vi "facade.vi"(0 "Data In":T13, 2 "Display State In":T3={"current frame index"=0, "number of images"=0, "ROI (frames)"={"ROI"=[]}, "control refs"={"frame"=refnum, "image"=refnum, "saveROIsButton"=refnum, "loadImageSwitch"=refnum, "loadROIsSwitch"=refnum, "saveROIsSwitch"=refnum, "loadImagePath"=refnum, "loadROIPath"=refnum, "redraw"=refnum}, "calibration"={"x"=0.0, "y"=0.0, "x unit"=enum."um", "y unit"=enum."um"}, "xpaths"={"x offset"="", "y offset"="", "z offset"=""}, "offset"=refnum, "XML description"="", "number of ROIs"=0.0, "ROI Tool Buttons Visible"={"Zoom Tool"=FALSE, "Selection Tool"=FALSE, "Pan Tool"=FALSE, "Point Tool"=FALSE, "Line Tool"=FALSE, "Rectangle Tool"=FALSE, "Rotated Rectangle Tool"=FALSE, "Polyline Tool"=FALSE, "Polygon Tool"=FALSE, "Freehand Tool"=FALSE, "Closed Freehand Tool"=FALSE, "Ellipse Tool"=FALSE, "Annulus Tool"=FALSE}, "ROI color"=0, "enable ROI numbering?"=FALSE, "selected path to save ROIs"=path "", "starting path"=path "", "loaded image path"=path "", "array of overlays"=[], "pointCollection"=refnum, "ROImode"=enum."IMAQROIs", "selected point ID"=0.0, "point radius"=0, "point colours"=[], "PlotAreaSize"={"Width"=0, "Height"=0}, "last action"=enum."not specified"} {"array of overlays"."overlay size" min=1}, 3 "Container State":T12, 5 "error in (no error)":errorcluster) -> (4 "error out":errorcluster, 6 "Data Out":T13, 7 "Display State Out":T3={"current frame index"=0, "number of images"=0, "ROI (frames)"={"ROI"=[]}, "control refs"={"frame"=refnum, "image"=refnum, "saveROIsButton"=refnum, "loadImageSwitch"=refnum, "loadROIsSwitch"=refnum, "saveROIsSwitch"=refnum, "loadImagePath"=refnum, "loadROIPath"=refnum, "redraw"=refnum}, "calibration"={"x"=0.0, "y"=0.0, "x unit"=enum."um", "y unit"=enum."um"}, "xpaths"={"x offset"="", "y offset"="", "z offset"=""}, "offset"=refnum, "XML description"="", "number of ROIs"=0.0, "ROI Tool Buttons Visible"={"Zoom Tool"=FALSE, "Selection Tool"=FALSE, "Pan Tool"=FALSE, "Point Tool"=FALSE, "Line Tool"=FALSE, "Rectangle Tool"=FALSE, "Rotated Rectangle Tool"=FALSE, "Polyline Tool"=FALSE, "Polygon Tool"=FALSE, "Freehand Tool"=FALSE, "Closed Freehand Tool"=FALSE, "Ellipse Tool"=FALSE, "Annulus Tool"=FALSE}, "ROI color"=0, "enable ROI numbering?"=FALSE, "selected path to save ROIs"=path "", "starting path"=path "", "loaded image path"=path "", "array of overlays"=[], "pointCollection"=refnum, "ROImode"=enum."IMAQROIs", "selected point ID"=0.0, "point radius"=0, "point colours"=[], "PlotAreaSize"={"Width"=0, "Height"=0}, "last action"=enum."not specified"} {"array of overlays"."overlay size" min=1}, 8 "Action":T2)   [LabVIEW 2010, in "XImage.xctl"]
uses:
  XImage.xctl
  data.ctl
  classes/ImageCollection/ImageCollection/ImageCollection.lvclass
  <vilib>/_xctls/Container State.ctl
  state.ctl
  classes/SpaceVector/SpaceVector/SpaceVector.lvclass
  classes/PointCollection/PointCollection/PointCollection.lvclass
  ROI_frames_cluster.ctl
  control_refs_cluster.ctl
  calibration_cluster.ctl
  enumerations/unit.ctl
  xpath_cluster.ctl
  overlays_cluster.ctl
  ROI_mode_enum.ctl
  last_action_enum.ctl
  <vilib>/_xctls/Action.ctl
  classes/Image/Image/Image.lvclass
  <vilib>/vision/Image Controls.llb/IMAQ Image.ctl
  <vilib>/Utility/inputDevices.llb/keyboardAcquire.vi
  <vilib>/Utility/inputDevices.llb/closeKeyboard.vi
  <vilib>/_xctls/XControlSupport.lvlib
panel:
  out "event case no.":i32
  in  "redraw":bool
  in  "savePointsButton":bool
  in  "loadPointsButton":bool
  in  "showHeaderButton":bool
  in  "loadROIPath":path caption="start path"
  in  "loadImagePath":path
  in  "loadROIsSwitch":bool=TRUE
  in  "saveROIsSwitch":bool=TRUE
  in  "loadImageSwitch":bool=TRUE
  out "progress bar":u8(slide) scale=0.0..100.0
  in  "loadROIsButton":bool
  in  "saveROIsButton":bool
  in  "loadImageButton":bool
  in  "frame":i32(slide) scale=0.0..10.0
  out "Image":T1(plugin-control)
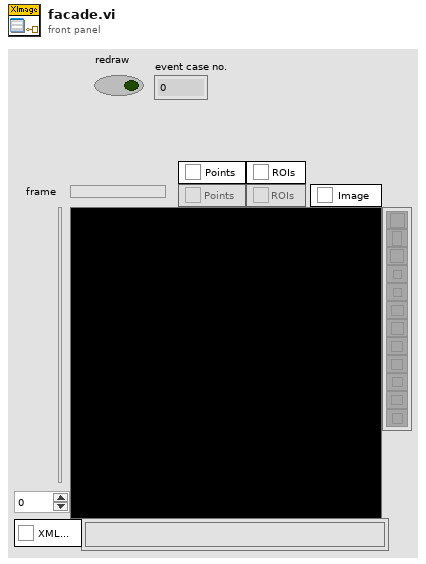
[diagram p1: front panel]
types:
  T1 = typedef "IMAQ Image.ctl" = refnum<image>
  T2 = typedef "XControlSupport.lvlib/Action.ctl" = cluster{"Data Changed?":bool, "State Changed?":bool, "Action Name":string}
  T3 = typedef "XImage.xctl/state.ctl" = cluster{"current frame index":i32, "number of images":i32, "ROI (frames)":T4, "control refs":T5, "calibration":T6, "xpaths":T8, "offset":refnum<class "SpaceVector.lvclass">, "XML description":string, "number of ROIs":dbl, "ROI Tool Buttons Visible":cluster{"Zoom Tool":bool, "Selection Tool":bool, "Pan Tool":bool, "Point Tool":bool, "Line Tool":bool, "Rectangle Tool":bool, "Rotated Rectangle Tool":bool, "Polyline Tool":bool, "Polygon Tool":bool, "Freehand Tool":bool, "Closed Freehand Tool":bool, "Ellipse Tool":bool, "Annulus Tool":bool}, "ROI color":u32, "enable ROI numbering?":bool, "selected path to save ROIs":path, "starting path":path, "loaded image path":path, "array of overlays":T9[], "pointCollection":refnum<class "PointCollection.lvclass">, "ROImode":T10, "selected point ID":dbl, "point radius":i32, "point colours":u32[], "PlotAreaSize":cluster{"Width":u32, "Height":u32}, "last action":T11}
  T4 = typedef "XImage.xctl/ROI_frames_cluster.ctl" = cluster{"ROI":cluster{"Global Rectangle":i32[], "Contours":cluster{"Contour Type":u32, "ROI Type":u32, "Points":i32[]}[]}[]}
  T5 = typedef "XImage.xctl/control_refs_cluster.ctl" = cluster{"frame":refnum<vi>, "image":refnum<vi>, "saveROIsButton":refnum<vi>, "loadImageSwitch":refnum<vi>, "loadROIsSwitch":refnum<vi>, "saveROIsSwitch":refnum<vi>, "loadImagePath":refnum<vi>, "loadROIPath":refnum<vi>, "redraw":refnum<vi>}
  T6 = typedef "XImage.xctl/calibration_cluster.ctl" = cluster{"x":dbl, "y":dbl, "x unit":T7, "y unit":T7}
  T7 = typedef "Image.lvclass/unit.ctl" = enum16{"um", "s"}
  T8 = typedef "XImage.xctl/xpath_cluster.ctl" = cluster{"x offset":string, "y offset":string, "z offset":string}
  T9 = typedef "XImage.xctl/overlays_cluster.ctl" = cluster{"overlay array":cluster{i32[][]}[], "overlay name":string, "color (red)":u32, "overlay size":i32, "overlay type":enum16{"crosshair", "circle"}}
  T10 = typedef "XImage.xctl/ROI_mode_enum.ctl" = enum16{"none", "IMAQROIs", "PointCollection"}
  T11 = typedef "XImage.xctl/last_action_enum.ctl" = enum16{"not specified", "image loaded", "frame changed", "ROIs changed"}
  T12 = typedef "XControlSupport.lvlib/Container State.ctl" = cluster{"Indicator?":bool, "Run Mode?":bool, " Refnum":refnum<vi>}
  T13 = typedef "XImage.xctl/data.ctl" = refnum<class "ImageCollection.lvclass">
  T14 = enum16{"0", "1", "2", "3", "4", "5", "6", "7", "8", "9", "A", "B", "C", "D", "E", "F", "G", "H", "I", "J", "K", "L", "M", "N", "O", "P", "Q", "R", "S", "T", "U", "V", "W", "X", "Y", "Z", "F1", "F2", "F3", "F4", "F5", "F6", "F7", "F8", "F9", "F10", "F11", "F12", "F13", "F14", "F15", "ADD", "BACK", "BACKSLASH", "CAPITAL", "COMMA", "DECIMAL", "DELETE", "DIVIDE", "DOWN", "END", "EQUALS", "ESCAPE", "GRAVE (`)", "HOME", "INSERT", "LBRACKET", "LCONTROL", "LEFT", "L ALT", "LSHIFT", "LWIN", "MINUS", "MULTIPLY", "NEXT", "NUMLOCK", "NUMPAD_0", "NUMPAD_1", "NUMPAD_2", "NUMPAD_3", "NUMPAD_4", "NUMPAD_5", "NUMPAD_6", "NUMPAD_7", "NUMPAD_8", "NUMPAD_9", "PAUSE", "PERIOD", "PRIOR (PG UP)", "RBRACKET", "RCONTROL", "RETURN", "RIGHT", "R ALT", "RSHIFT", "RWIN", "SCROLL", "SEMICOLON", "SLASH", "SPACE", "SUBTRACT", "TAB", "UP", "ENTER (num pad)", "' (quote)"}
  T15 = cluster{"Zoom Tool":bool, "Selection Tool":bool, "Pan Tool":bool, "Point Tool":bool, "Line Tool":bool, "Rectangle Tool":bool, "Rotated Rectangle Tool":bool, "Polyline Tool":bool, "Polygon Tool":bool, "Freehand Tool":bool, "Closed Freehand Tool":bool, "Ellipse Tool":bool, "Annulus Tool":bool}
  T16 = cluster{"Global Rectangle":i32[], "Contours":cluster{"Contour Type":u32, "ROI Type":u32, "Points":i32[]}[]}
  T17 = cluster{"Global Rectangle":i32[], "Contours":cluster{"Contour Type":u32, "ROI Type":u32, "Points":i32[]}[]}[]
  T18 = cluster{"Contour Type":u32, "ROI Type":u32, "Points":i32[]}[]
  T19 = enum8{"Enabled", "Disabled", "Disabled and Grayed Out"}
  T20 = typedef "Image Type" = u32
  T21 = enum16{"0", "1", "2", "3", "4", "5", "6", "7", "8", "9", "A", "B", "C", "D", "E", "F", "G", "H", "I", "J", "K", "L", "M", "N", "O", "P", "Q", "R", "S", "T", "U", "V", "W", "X", "Y", "Z", "F1", "F2", "F3", "F4", "F5", "F6", "F7", "F8", "F9", "F10", "F11", "F12", "F13", "F14", "F15", "ADD", "BACK", "BACKSLASH", "CAPITAL", "COMMA", "DECIMAL", "DELETE", "DIVIDE", "DOWN", "END", "EQUALS", "ESCAPE", "GRAVE (`)", "HOME", "INSERT", "LBRACKET", "LCONTROL", "LEFT", "L ALT", "LSHIFT", "LWIN", "MINUS", "MULTIPLY", "NEXT", "NUMLOCK", "NUMPAD_0", "NUMPAD_1", "NUMPAD_2", "NUMPAD_3", "NUMPAD_4", "NUMPAD_5", "NUMPAD_6", "NUMPAD_7", "NUMPAD_8", "NUMPAD_9", "PAUSE", "PERIOD", "PRIOR (PG UP)", "RBRACKET", "RCONTROL", "RETURN", "RIGHT", "R ALT", "RSHIFT", "RWIN", "SCROLL", "SEMICOLON", "SLASH", "SPACE", "SUBTRACT", "TAB", "UP", "ENTER (num pad)", "' (quote)"}[]
  T22 = typedef "LVRectTypeDef.ctl" = cluster{"left":i16, "top":i16, "right":i16, "bottom":i16}
  T23 = typedef "LVBoundsTypeDef.ctl" = cluster{"Width":u32, "Height":u32}
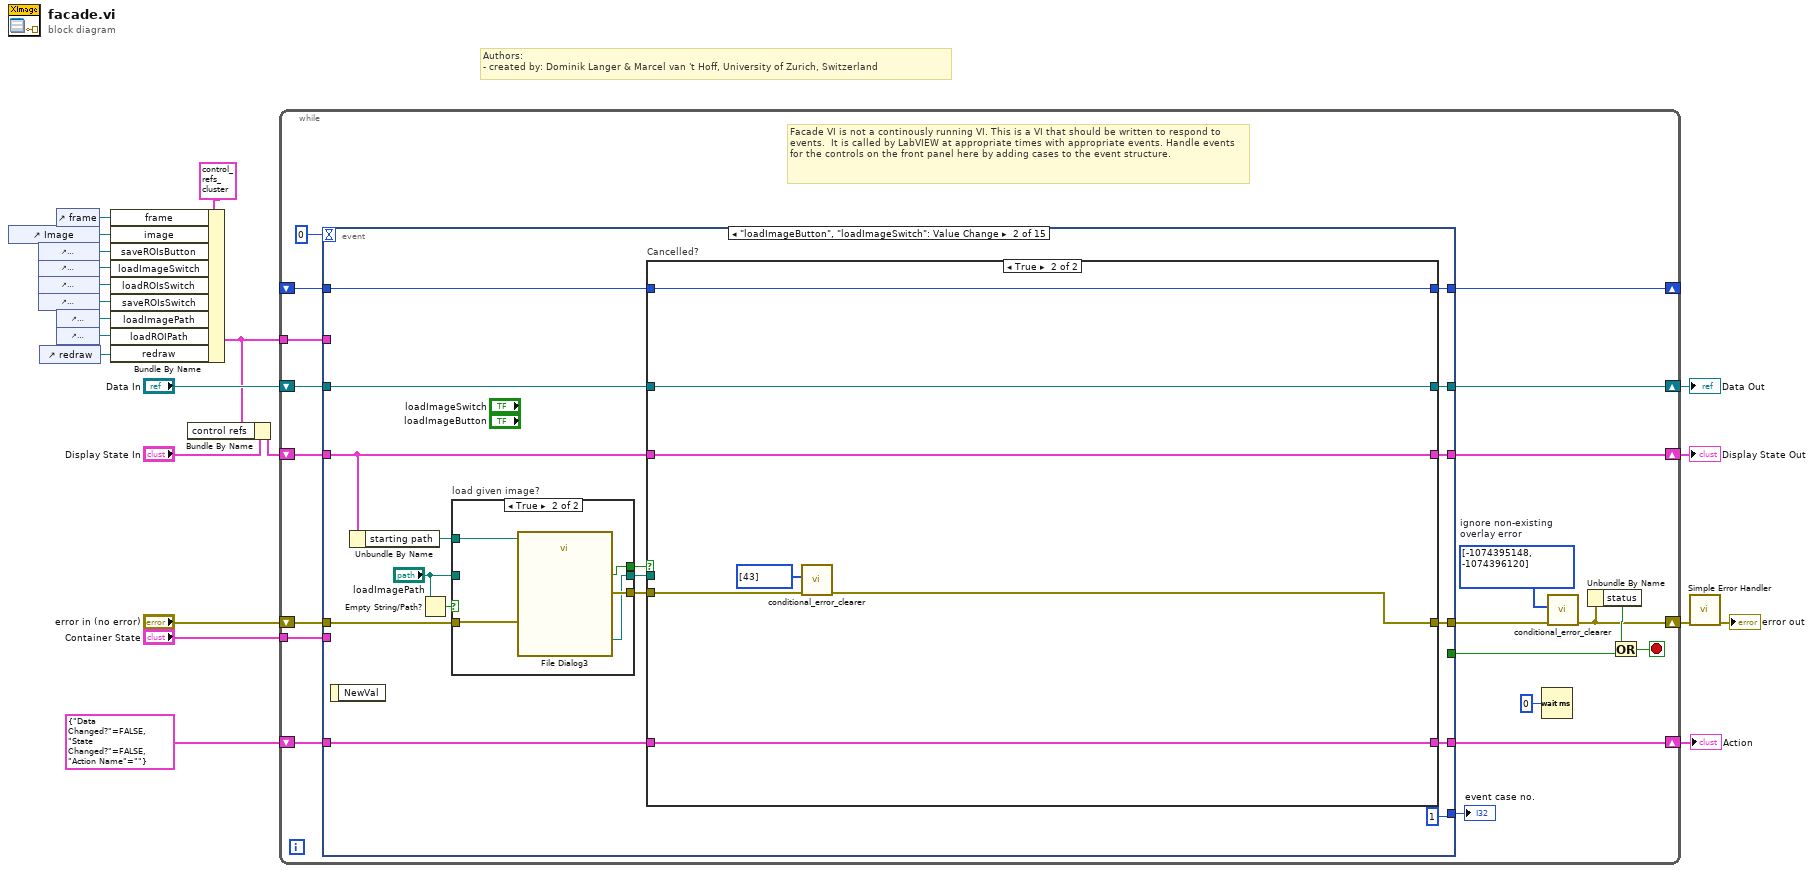
[diagram p0: block diagram]
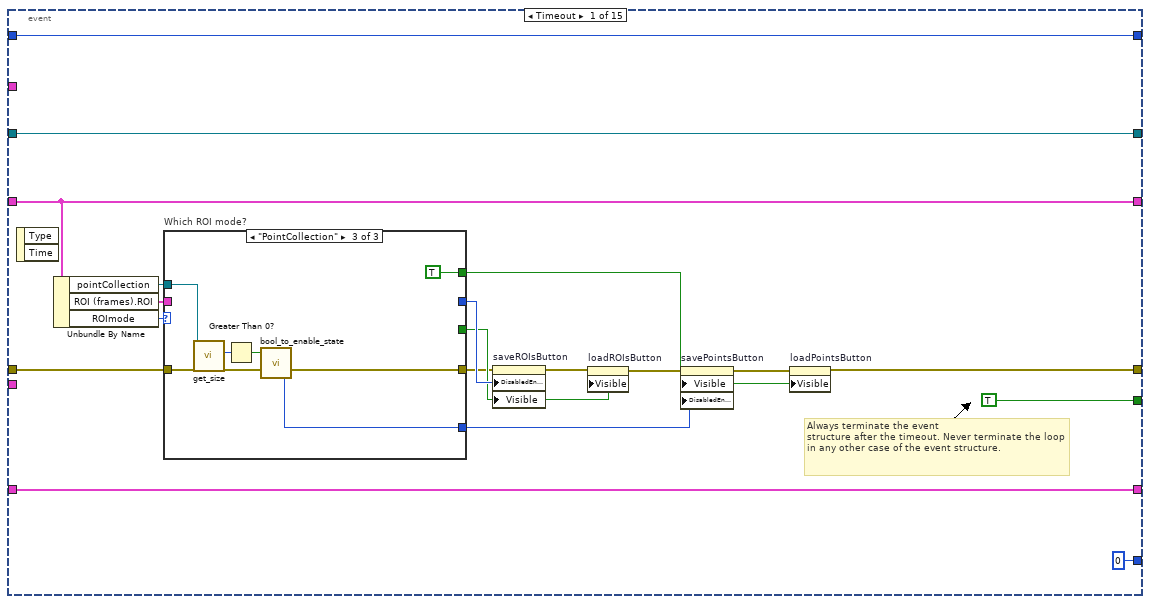
[diagram p2: hidden frame]
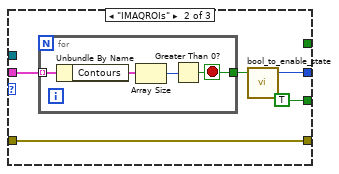
[diagram p4: hidden frame]
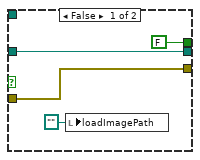
[diagram p5: hidden frame]
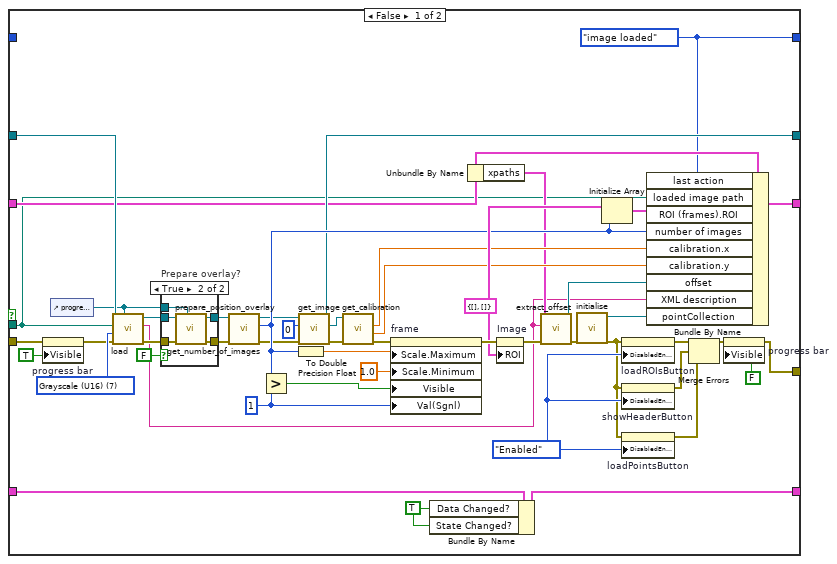
[diagram p6: hidden frame]
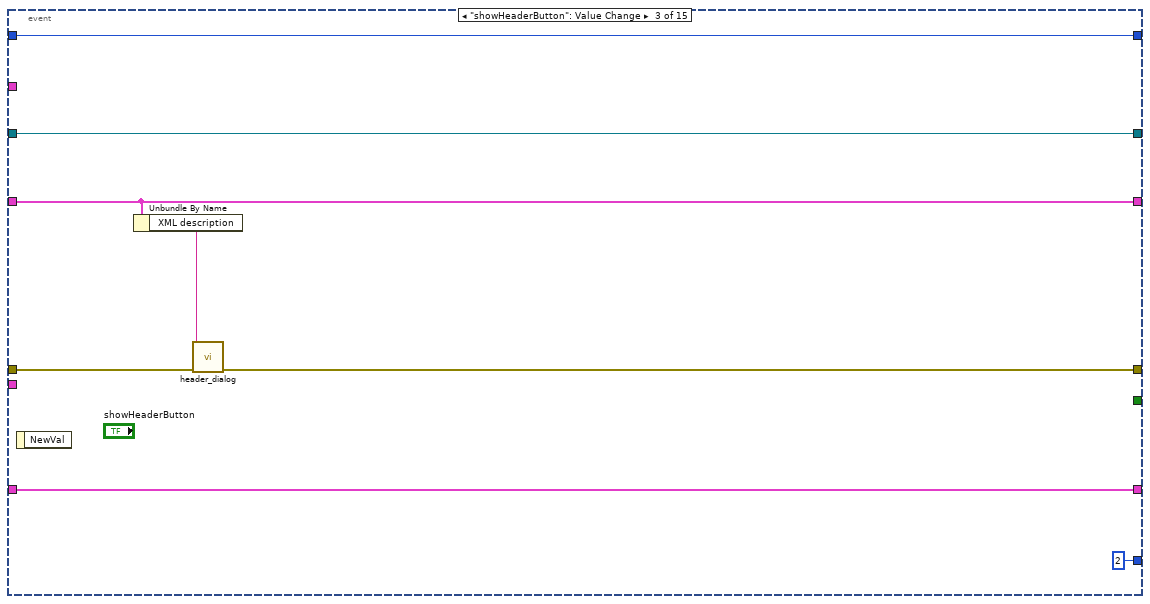
[diagram p8: hidden frame]
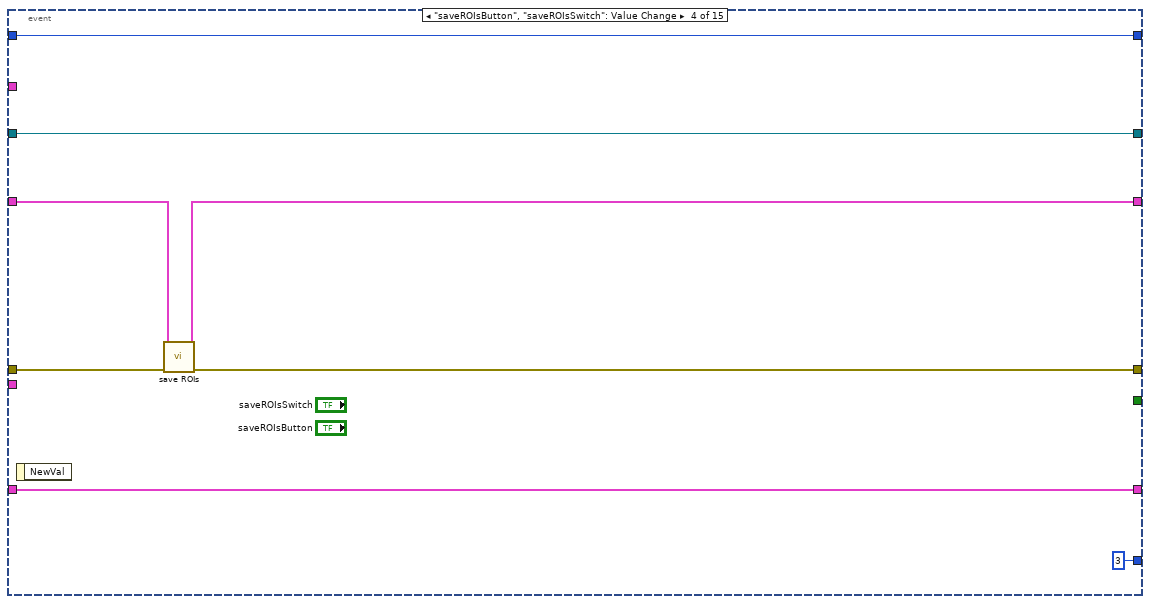
[diagram p9: hidden frame]
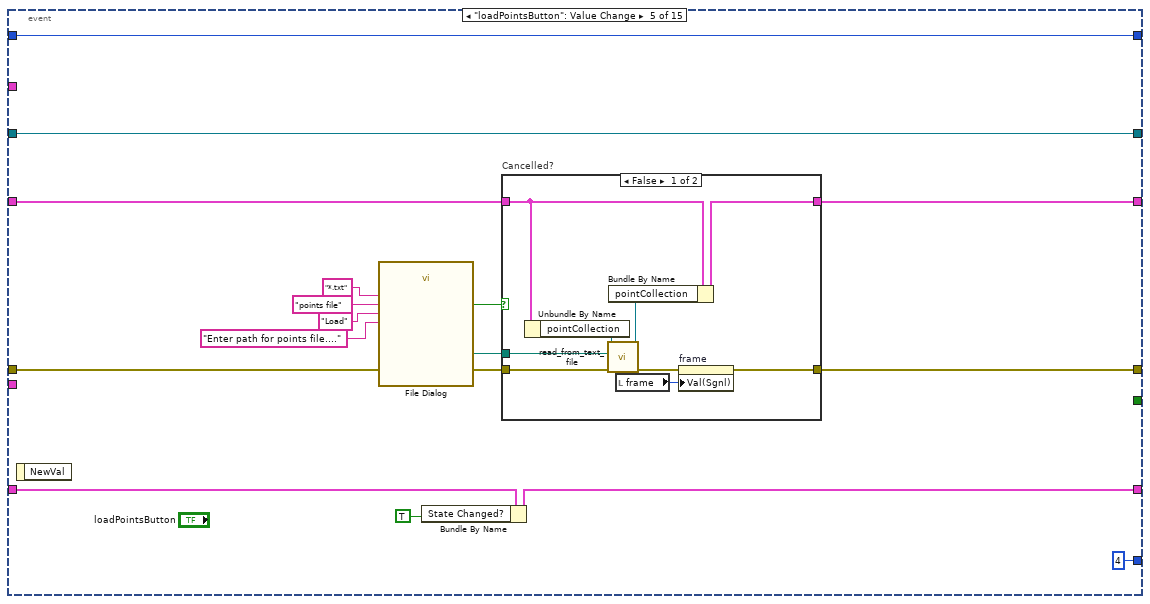
[diagram p10: hidden frame]
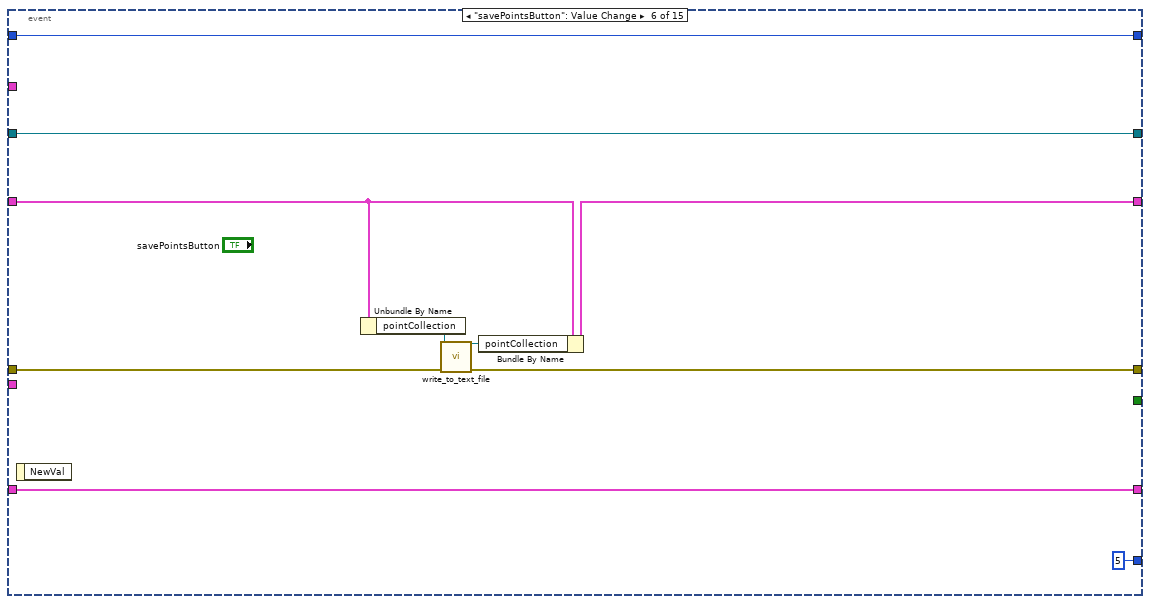
[diagram p12: hidden frame]
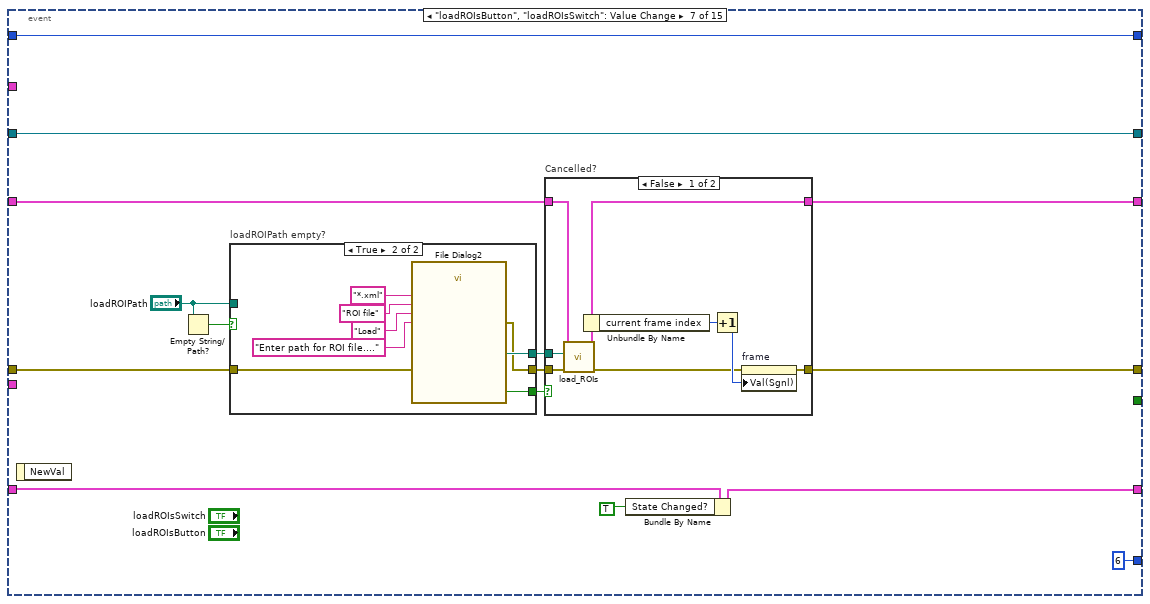
[diagram p13: hidden frame]
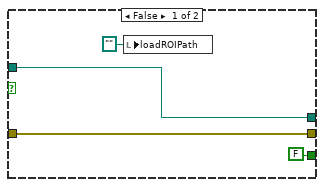
[diagram p14: hidden frame]
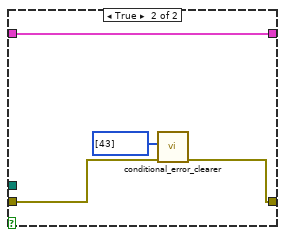
[diagram p15: hidden frame]
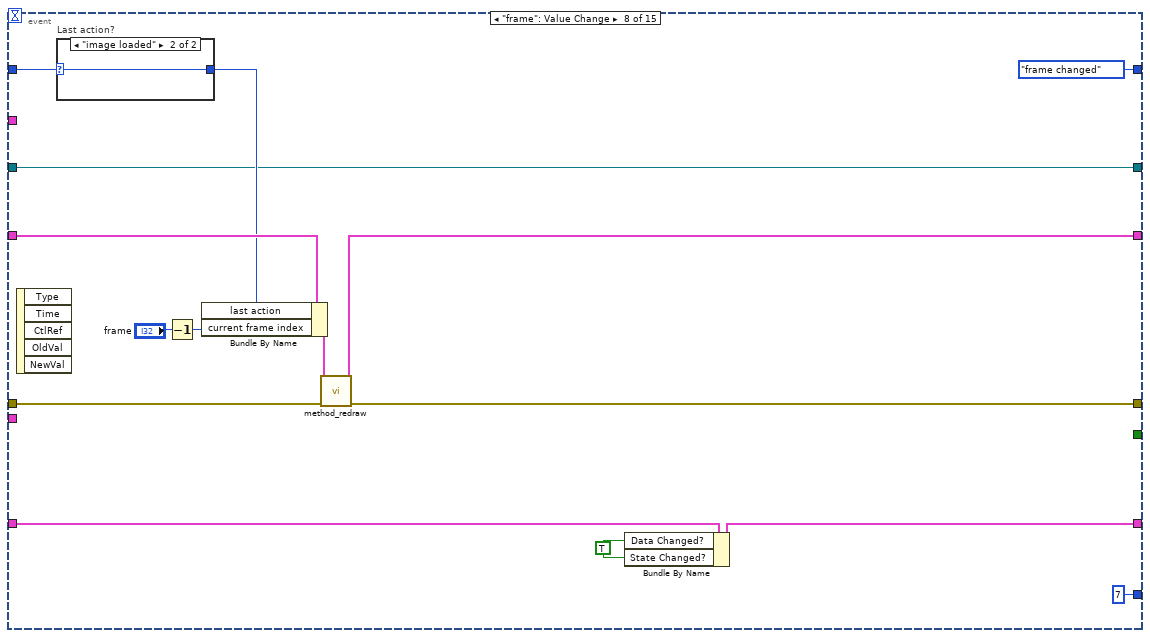
[diagram p16: hidden frame]
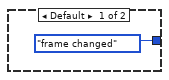
[diagram p17: hidden frame]
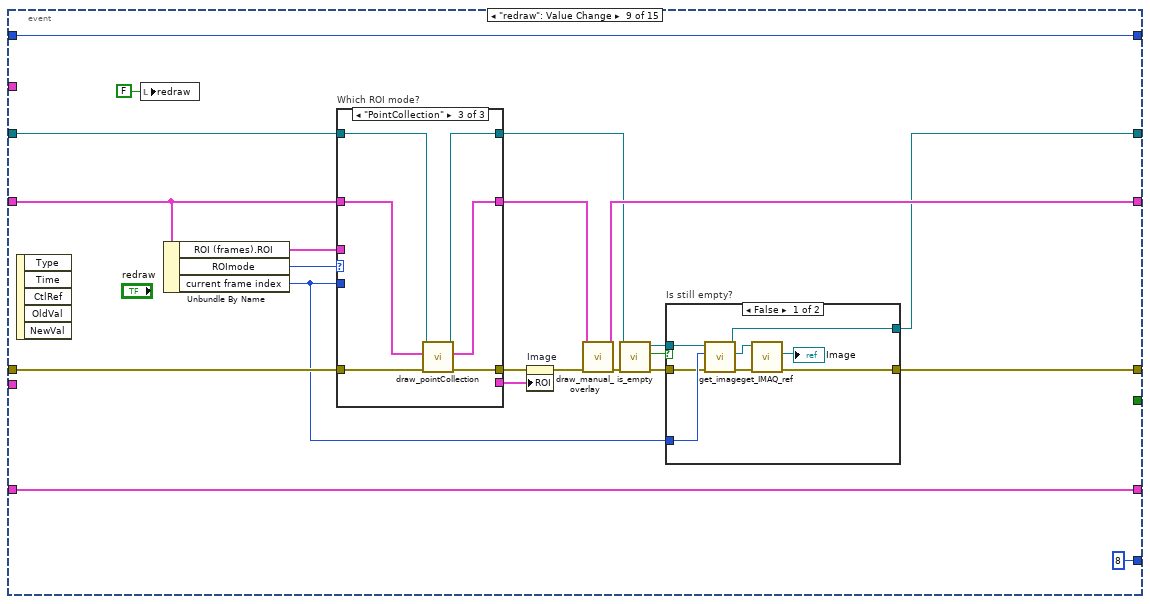
[diagram p18: hidden frame]
diagram:
  # "Authors: \n- created by: Dominik Langer & Marcel van 't Hoff, University of Zurich, Switzerland"
  n1 = control-ref of="Image"() -> (w8:refnum<vi>)
  n2 = control-ref of="saveROIsButton"() -> (w9:refnum<vi>)
  n3 = control-ref of="loadImageSwitch"() -> (w10:refnum<vi>)
  n4 = control-ref of="loadROIsSwitch"() -> (w11:refnum<vi>)
  n5 = control-ref of="saveROIsSwitch"() -> (w12:refnum<vi>)
  n6 = control-ref of="redraw"() -> (w6:refnum<vi>)
  n7 = control-ref of="frame"() -> (w7:refnum<vi>)
  n8 = control-ref of="loadImagePath"() -> (w13:refnum<vi>)
  n9 = control-ref of="loadROIPath"() -> (w5:refnum<vi>)
  n10 = Bundle By Name(cluster=T5 {"frame"=refnum, "image"=refnum, "saveROIsButton"=refnum, "loadImageSwitch"=refnum, "loadROIsSwitch"=refnum, "saveROIsSwitch"=refnum, "loadImagePath"=refnum, "loadROIPath"=refnum, "redraw"=refnum} ("control refs"), "frame"=w7, "image"=w8, "saveROIsButton"=w9, "loadImageSwitch"=w10, "loadROIsSwitch"=w11, "saveROIsSwitch"=w12, "loadImagePath"=w13, "loadROIPath"=w5, "redraw"=w6) -> (w1:T5)
  n11 = Bundle By Name(cluster="Display State In", "control refs"=w1) -> (w2:T3)
  n12 = while {
    shift-right: [w42] -> w19
    shift-left: w2 -> [w26]
    tunnel: "Container State" -> [w40]
    shift-right: [w38] -> w22
    shift-left: "Data In" -> [w39]
    shift-right: [w32] -> w18
    shift-left: T2 {"Data Changed?"=FALSE, "State Changed?"=FALSE, "Action Name"=""} ("Action") -> [w37]
    shift-right: [w31] -> w15
    shift-left: "error in (no error)" -> [w36]
    shift-right: [w28] -> _
    shift-left: _ -> [w27]
    tunnel: w1 -> [w23]
    stop <- w34 stop-if-true
    w29 = i32[] [-1074395148, -1074396120]  # ignore non-existing overlay error
    # "Facade VI is not a continously running VI. This is a VI that should be written to respond to events.  It is called by LabVIEW at appropriate times with appropriate events. Handle events for the controls on the front panel here by adding cases to the event structure."
    n13 = event shown="[1] \"loadImageButton\", \"loadImageSwitch\": Value Change" {
      selector: _ -> [_ _ _ _ _ _ _ _ _ _ _ _ _ _ _]
      dyn-events: _ -> [_ _ _ _ _ _ _ _ _ _ _ _ _ _ _]
      timeout: 0 -> [_ _ _ _ _ _ _ _ _ _ _ _ _ _ _]
      tunnel: w26 -> [w58 w83 w173 w178 w198 w215 w230 w271 w292 w339 w469 w479 w512 w521 _]
      tunnel: [w58 w92 w173 w181 w197 w214 w234 w263 w288 w328 w468 w477 w512 w520 w608] -> w42
      tunnel: [TRUE _ _ _ _ _ _ _ _ _ _ _ _ _ _] -> w35
      tunnel: w40 -> [_ _ _ _ _ _ _ _ _ _ _ w497 w513 w525 w609]
      tunnel: w39 -> [w60 w93 w175 w183 w199 w217 w235 w261 w286 w332 w471 w481 w511 w577 w581]
      tunnel: [w60 w91 w175 w183 w199 w217 w235 w261 w282 w333 w470 w481 w511 w577 T13 refnum ("imageCollection")] -> w38
      tunnel: [w59 w94 w174 w182 w194 w220 w232 w272 w298 w335 w466 w498 w510 w516 w605] -> w32
      tunnel: w37 -> [w59 w95 w174 w182 w195 w220 w233 w273 w298 w336 w467 w498 w510 w517 w606]
      tunnel: w36 -> [w46 w87 w171 w179 w188 w219 w226 w260 w285 w337 w465 w495 w507 w524 w580]
      tunnel: [w48 w86 w170 w180 w193 w218 w225 w262 w283 w330 w464 w478 w506 w544 w592] -> w30
      tunnel: [w56 w81 w169 w177 w185 w212 w222 last_action_enum."frame changed" ("last action") w297 w334 w454 w483 w505 w515 w588] -> w28
      tunnel: w27 -> [w56 w80 w169 w177 w185 w212 w222 w268 w297 w334 w454 w483 w505 w515 w588]
      tunnel: [0 1 2 3 4 5 6 7 8 9 10 11 12 13 14] -> w25
      tunnel: w23 -> [_ _ _ _ _ _ _ _ _ _ _ _ _ _ w585]
      event Timeout {
        # "Always terminate the event\nstructure after the timeout. Never terminate the loop in any other case of the event structure."
        n14 = event-data() -> ()  [unwired: 1 in, 2 out]
        n15 = Unbundle By Name(w58) -> ("pointCollection"=w47:refnum<class "PointCollection.lvclass">, "ROI (frames).ROI"=w57:T17, "ROImode"=w55:T10)
        n16 = case "Which ROI mode?" shown="\"PointCollection\"" w55 {
          tunnel: w57 -> [_ w67 _]
          tunnel: [_ w65 _] -> w54
          tunnel: [_ TRUE _] -> w52
          tunnel: [_ _ TRUE] -> w49
          tunnel: w47 -> [_ _ w76]
          tunnel: w46 -> [w62 w63 w77]
          tunnel: [w62 w63 w75] -> w45
          tunnel: [_ _ w72] -> w44
          frame "none", Default {
          }
          frame "IMAQROIs" {
            n17 = for {
              tunnel: w67 -> [w71] mode=indexing
              tunnel: [w68] -> w66
              stop <- w68 stop-if-true
              n18 = Unbundle By Name(w71) -> ("Contours"=w70:T18)
              n19 = Array Size(array=w70) -> (size(s)=w69:i32)
              n20 = Greater Than 0?(x=w69) -> (x > 0?=w68:bool)
            }
            n21 = call "bool_to_enable_state.vi"("boolean in"=w66) -> ("enabled status out"=w65:T19)  [unwired: 4 in]
          }
          frame "PointCollection" {
            n22 = call "get_size.vi"("error in (no error)"=w77, "PointCollection in"=w76) -> ("error out"=w75:errorcluster, "number of points"=w74:i32)  [unwired: 7 in, 1 out]
            n23 = Greater Than 0?(x=w74) -> (x > 0?=w73:bool)
            n24 = call "bool_to_enable_state.vi"("boolean in"=w73) -> ("enabled status out"=w72:T19)  [unwired: 4 in]
          }
        }
        n25 = property on="saveROIsButton" class="Bool"(error in=w45, "DisabledEnum"=w54, "Visible"=w52) -> (error out=w53:errorcluster)  [unwired: 1 in, 1 out]
        n26 = property on="loadROIsButton" class="Bool"(error in=w53, "Visible"=w52) -> (error out=w51:errorcluster)  [unwired: 1 in, 1 out]
        n27 = property on="savePointsButton" class="Bool"(error in=w51, "Visible"=w49, "DisabledEnum"=w44) -> (error out=w50:errorcluster)  [unwired: 1 in, 1 out]
        n28 = property on="loadPointsButton" class="Bool"(error in=w50, "Visible"=w49) -> (error out=w48:errorcluster)  [unwired: 1 in, 1 out]
      }
      event "loadImageButton", "loadImageSwitch": Value Change {
        n29 = event-data() -> ()  [unwired: 1 in, 1 out]
        n30 = Unbundle By Name(w83) -> ("starting path"=w82:path)
        n31 = Empty String/Path?(string/path="loadImagePath") -> (empty?=w85:bool)
        n32 = case "load given image?" shown="True" w85 {
          tunnel: [w98 w104] -> w90
          tunnel: [w99 w103] -> w89
          tunnel: [FALSE ("cancelled") w102] -> w88
          tunnel: w87 -> [w98 w101]
          tunnel: "loadImagePath" -> [w99 _]
          tunnel: w82 -> [_ w100]
          frame False {
            n33 = local write "loadImagePath"(path "") -> ()
          }
          frame True {
            n34 = call "File Dialog3"("start path"=w100, "error in"=w101) -> ("selected path"=w103:path, "cancelled"=w102:bool, "error out"=w104:errorcluster)  [unwired: 10 in, 1 out]
          }
        }
        n35 = case "Cancelled?" shown="True" w88 {
          tunnel: w95 -> [w150 w165]
          tunnel: [w149 w165] -> w94
          tunnel: w93 -> [w147 w167]
          tunnel: w83 -> [w125 w166]
          tunnel: [w145 w166] -> w92
          tunnel: [w130 w167] -> w91
          tunnel: w90 -> [w139 w164]
          tunnel: w89 -> [w105 _]
          tunnel: [w123 w163] -> w86
          tunnel: [w106 w161] -> w81
          tunnel: w80 -> [_ w161]
          frame False {
            w106 = last_action_enum."image loaded" ("last action")
            w111 = T19."Enabled" ("Disabled")
            w142 = T16 {"Global Rectangle"=[], "Contours"=[]} ("ROI")
            w146 = T20 7 items=["Grayscale (U8)", "Grayscale (I16)", "Grayscale (SGL)", "Complex (CSG)", "RGB (U32)", "HSL (U32)", "RGB (U64)", "Grayscale (U16)"] ("Image Type")
            w107 = TRUE ("Data Changed?")
            w148 = 1 ("y")
            n36 = property on="progress bar" class="Slide (strict)"(error in=w139, "Visible"=TRUE) -> (error out=w138:errorcluster)  [unwired: 1 in, 1 out]
            n37 = control-ref of="progress bar"() -> (w118:refnum<vi>)
            n38 = call "load.vi"("progress bar ref"=w118, "error in (no error)"=w138, "Image Type"=w146, "path in"=w105, "ImageCollection in"=w147) -> ("error out"=w122:errorcluster, "description"=w117:string, "ImageCollection out"=w120:T13)  [unwired: 2 in, 2 out]
            n39 = case "Prepare overlay?" shown="True" FALSE {
              tunnel: w122 -> [w155 w160]
              tunnel: [w155 w159] -> w121
              tunnel: w120 -> [w154 w158]
              tunnel: [w154 w157] -> w119
              tunnel: w118 -> [_ w156]
              frame False {
              }
              frame True {
                n40 = call "prepare_position_overlay.vi"("progress bar ref"=w156, "error in (no error)"=w160, "ImageCollection in"=w158) -> ("error out"=w159:errorcluster, "ImageCollection out"=w157:T13)  [unwired: 6 in, 1 out]
              }
            }
            n41 = call-dynamic "get_number_of_images.vi"("error in (no error)"=w121, "ImageCollection in"=w119) -> ("error out"=w133:errorcluster, "size"=w141:i32, "ImageCollection out"=w131:T13)  [unwired: 7 in]
            n42 = Greater?(x=w141, y=w148) -> (0:w151:bool)
            n43 = To Double Precision Float(number=w141) -> (double precision float=w153:dbl)
            n44 = call-dynamic "get_image.vi"("error in (no error)"=w133, "index"=0, "ImageCollection in"=w131) -> ("error out"=w136:errorcluster, "Image.lvclass"=w135:refnum<class "Image.lvclass">, "ImageCollection out"=w130:T13)  [unwired: 6 in]
            n45 = call "get_calibration.vi"("error in (no error)"=w136, "Image.lvclass in"=w135) -> ("error out"=w132:errorcluster, "y"=w128:dbl, "x"=w129:dbl)  [unwired: 4 in, 3 out]
            n46 = property on="frame" class="Slide (strict)"(error in=w132, "Scale.Maximum"=w153, "Scale.Minimum"=1.0 ("Scale.Range:Minimum"), "Visible"=w151, "Val(Sgnl)"=w148) -> (error out=w143:errorcluster)  [unwired: 1 in, 1 out]
            n47 = Bundle By Name(cluster=w150, "Data Changed?"=w107, "State Changed?"=w107) -> (w149:T2)
            n48 = Unbundle By Name(w125) -> ("xpaths"=w124:T8)
            n49 = property on="Image" class="ImageControl"(error in=w143, "ROI"=w142) -> (error out=w127:errorcluster)  [unwired: 1 in, 1 out]
            n50 = call "extract_offset.vi"("error in (no error)"=w127, "xml header string"=w117, "xpaths"=w124) -> ("error out"=w110:errorcluster, "offset"=w126:refnum<class "SpaceVector.lvclass">)  [unwired: 7 in]
            n51 = call "initialise.vi"("error in (no error)"=w110) -> ("error out"=w109:errorcluster, "PointCollection out"=w108:refnum<class "PointCollection.lvclass">)  [unwired: 9 in]
            n52 = Initialize Array(w142, w141) -> (w144:T17)
            n53 = property on="loadROIsButton" class="Bool"(error in=w109, "DisabledEnum"=w111) -> (error out=w115:errorcluster)  [unwired: 1 in, 1 out]
            n54 = property on="showHeaderButton" class="Bool"(error in=w109, "DisabledEnum"=w111) -> (error out=w112:errorcluster)  [unwired: 1 in, 1 out]
            n55 = property on="loadPointsButton" class="Bool"(error in=w109, "DisabledEnum"=w111) -> (error out=w113:errorcluster)  [unwired: 1 in, 1 out]
            n56 = Bundle By Name(cluster=w125, "last action"=w106, "loaded image path"=w105, "ROI (frames).ROI"=w144, "number of images"=w141, "calibration.x"=w129, "calibration.y"=w128, "offset"=w126, "XML description"=w117, "pointCollection"=w108) -> (w145:T3)
            n57 = Merge Errors(w115, w112, w113) -> (w114:errorcluster)
            n58 = property on="progress bar" class="Slide (strict)"(error in=w114, "Visible"=FALSE) -> (error out=w123:errorcluster)  [unwired: 1 in, 1 out]
          }
          frame True {
            n59 = call "conditional_error_clearer.vi"("error in (no error)"=w164, "array of clearable error codes"=i32[] [43]) -> ("error out"=w163:errorcluster)  [unwired: 9 in]
          }
        }
      }
      event "showHeaderButton": Value Change {
        n60 = event-data() -> ()  [unwired: 1 in, 1 out]
        n61 = Unbundle By Name(w173) -> ("XML description"=w172:string)
        n62 = call "header_dialog.vi"("error in (no error)"=w171, "header string in"=w172) -> ("error out"=w170:errorcluster)  [unwired: 9 in]
      }
      event "saveROIsButton", "saveROIsSwitch": Value Change {
        n63 = event-data() -> ()  [unwired: 1 in, 1 out]
        n64 = call "save ROIs.vi"("error out"=w179, "Display State in"=w178) -> ("error out"=w180:errorcluster, "Display State out"=w181:T3)  [unwired: 7 in, 1 out]
      }
      event "loadPointsButton": Value Change {
        n65 = event-data() -> ()  [unwired: 1 in, 1 out]
        n66 = call "File Dialog"("prompt"="Enter path for points file....", "button label"="Load", "error in"=w188, "pattern (all files)"="*.txt", "pattern label"="points file") -> ("selected path"=w187:path, "cancelled"=w186:bool)  [unwired: 7 in, 2 out]
        n67 = Bundle By Name(cluster=w195, "State Changed?"=TRUE) -> (w194:T2)
        n68 = case "Cancelled?" shown="False" w186 {
          tunnel: w198 -> [w206 w210]
          tunnel: [w205 w210] -> w197
          tunnel: [w203 w209] -> w193
          tunnel: w188 -> [w201 w209]
          tunnel: w187 -> [w200 _]
          frame False {
            n69 = Unbundle By Name(w206) -> ("pointCollection"=w207:refnum<class "PointCollection.lvclass">)
            n70 = call "read_from_text_file.vi"("error in (no error)"=w201, "file (use dialog)"=w200, "PointCollection in"=w207) -> ("error out"=w204:errorcluster, "PointCollection out"=w208:refnum<class "PointCollection.lvclass">)  [unwired: 7 in]
            n71 = Bundle By Name(cluster=w206, "pointCollection"=w208) -> (w205:T3)
            n72 = local read "frame"() -> (w202:i32)
            n73 = property on="frame" class="Slide (strict)"(error in=w204, "Val(Sgnl)"=w202) -> (error out=w203:errorcluster)  [unwired: 1 in, 1 out]
          }
          frame True {
          }
        }
      }
      event "savePointsButton": Value Change {
        n74 = event-data() -> ()  [unwired: 1 in, 1 out]
        n75 = Unbundle By Name(w215) -> ("pointCollection"=w216:refnum<class "PointCollection.lvclass">)
        n76 = call "write_to_text_file.vi"("error in (no error)"=w219, "PointCollection in"=w216) -> ("error out"=w218:errorcluster, "PointCollection out"=w213:refnum<class "PointCollection.lvclass">)  [unwired: 8 in]
        n77 = Bundle By Name(cluster=w215, "pointCollection"=w213) -> (w214:T3)
      }
      event "loadROIsButton", "loadROIsSwitch": Value Change {
        n78 = event-data() -> ()  [unwired: 1 in, 1 out]
        n79 = Empty String/Path?(string/path="loadROIPath") -> (empty?=w223:bool)
        n80 = case "loadROIPath empty?" shown="True" w223 {
          tunnel: [w237 w247] -> w229
          tunnel: [w239 w246] -> w228
          tunnel: [FALSE ("cancelled") w245] -> w227
          tunnel: w226 -> [w239 w240]
          tunnel: "loadROIPath" -> [w237 _]
          frame False {
            n81 = local write "loadROIPath"(path "") -> ()
          }
          frame True {
            n82 = call "File Dialog2"("prompt"="Enter path for ROI file....", "button label"="Load", "error in"=w240, "pattern (all files)"="*.xml", "pattern label"="ROI file") -> ("selected path"=w247:path, "cancelled"=w245:bool, "error out"=w246:errorcluster)  [unwired: 7 in, 1 out]
          }
        }
        n83 = case "Cancelled?" shown="False" w227 {
          tunnel: [w248 w259] -> w234
          tunnel: w230 -> [w250 w259]
          tunnel: w229 -> [w252 _]
          tunnel: w228 -> [w251 w257]
          tunnel: [w253 w256] -> w225
          frame False {
            n84 = call "load_ROIs.vi"("error in"=w251, "selected path"=w252, "Display State in"=w250) -> ("error out"=w249:errorcluster, "Display State out"=w248:T3)  [unwired: 7 in]
            n85 = Unbundle By Name(w248) -> ("current frame index"=w255:i32)
            n86 = Increment(x=w255) -> (x+1=w254:i32)
            n87 = property on="frame" class="Slide (strict)"(error in=w249, "Val(Sgnl)"=w254) -> (error out=w253:errorcluster)  [unwired: 1 in, 1 out]
          }
          frame True {
            n88 = call "conditional_error_clearer.vi"("error in (no error)"=w257, "array of clearable error codes"=i32[] [43]) -> ("error out"=w256:errorcluster)  [unwired: 9 in]
          }
        }
        n89 = Bundle By Name(cluster=w233, "State Changed?"=TRUE) -> (w232:T2)
      }
      event "frame": Value Change {
        w270 = TRUE ("State Changed?")
        n90 = event-data() -> ()  [unwired: 1 in, 5 out]
        n91 = case "Last action?" shown="\"image loaded\"" w268 {
          selector: w268 -> [_ w276]
          tunnel: [last_action_enum."frame changed" ("last action") w276] -> w267
          frame Default {
          }
          frame "image loaded" {
          }
        }
        n92 = Decrement(x="frame") -> (x-1=w269:i32)
        n93 = Bundle By Name(cluster=w271, "last action"=w267, "current frame index"=w269) -> (w264:T3)
        n94 = call "method_redraw.vi"("Display State In"=w264, "error in (no error)"=w260) -> ("Display State Out"=w263:T3, "error out"=w262:errorcluster)  [unwired: 12 in]
        n95 = Bundle By Name(cluster=w273, "Data Changed?"=w270, "State Changed?"=w270) -> (w272:T2)
      }
      event "redraw": Value Change {
        n96 = event-data() -> ()  [unwired: 1 in, 5 out]
        n97 = local write "redraw"(FALSE ("redraw")) -> ()
        n98 = Unbundle By Name(w292) -> ("ROI (frames).ROI"=w287:T17, "ROImode"=w293:T10, "current frame index"=w284:i32)
        n99 = case "Which ROI mode?" shown="\"PointCollection\"" w293 {
          tunnel: w292 -> [w310 w315 w320]
          tunnel: [w310 w314 w325] -> w289
          tunnel: w285 -> [w311 w317 w323]
          tunnel: [w311 w316 w322] -> w294
          tunnel: [w309 w318 w324] -> w277
          tunnel: [_ w319 _] -> w295
          tunnel: w286 -> [w309 w318 w321]
          tunnel: w284 -> [_ w313 _]
          tunnel: w287 -> [_ w312 _]
          frame "none", Default {
          }
          frame "IMAQROIs" {
            n100 = Index Array(array=w312, index=w313) -> (element=w319:T16)
            n101 = call "number_ROIs.vi"("error in"=w317, "Display State In"=w315) -> ("error out"=w316:errorcluster, "Display State Out"=w314:T3)  [unwired: 8 in]
          }
          frame "PointCollection" {
            n102 = call "draw_pointCollection.vi"("error in (no error)"=w323, "Display State In"=w320, "ImageCollection in"=w321) -> ("error out"=w322:errorcluster, "Display State Out"=w325:T3, "ImageCollection out"=w324:T13)  [unwired: 6 in]
          }
        }
        n103 = property on="Image" class="ImageControl"(error in=w294, "ROI"=w295) -> (error out=w290:errorcluster)  [unwired: 1 in, 1 out]
        n104 = call "draw_manual_overlay.vi"("error in"=w290, "Display State In"=w289) -> ("error out"=w281:errorcluster, "Display State Out"=w288:T3)  [unwired: 8 in]
        n105 = call "is_empty.vi"("error in (no error)"=w281, "ImageCollection in"=w277) -> ("error out"=w280:errorcluster, "is empty?"=w278:bool, "ImageCollection out"=w279:T13)  [unwired: 7 in]
        n106 = case "Is still empty?" shown="False" w278 {
          tunnel: w284 -> [w303 _]
          tunnel: [w302 w308] -> w283
          tunnel: [w301 w307] -> w282
          tunnel: w280 -> [w300 w308]
          tunnel: w279 -> [w299 w307]
          frame False {
            n107 = call-dynamic "get_image.vi"("error in (no error)"=w300, "index"=w303, "ImageCollection in"=w299) -> ("error out"=w306:errorcluster, "Image.lvclass"=w305:refnum<class "Image.lvclass">, "ImageCollection out"=w301:T13)  [unwired: 6 in]
            n108 = call-dynamic "get_IMAQ_ref.vi"("error in (no error)"=w306, "Image.lvclass in"=w305) -> ("error out"=w302:errorcluster, "Image"=→"Image":T1)  [unwired: 5 in, 3 out]
          }
          frame True {
          }
        }
      }
      event "Image": Mouse Up {
        n109 = event-data() -> ()  [unwired: 1 in, 1 out]
        n110 = Unbundle By Name(w339) -> ("ROImode"=w341:T10, "current frame index"=w343:i32, "ROI (frames).ROI"=w340:T17)
        n111 = invoke on="Image" class="ImageControl" method="Get Last Event"(error in=w337) -> (error out=w338:errorcluster, "Tool"=w348:i32, "Coordinates"=w345:i32[])  [unwired: 7 in, 5 out]
        n112 = Index Array(array=w345) -> (element #1=w347:i32, element #2=w344:i32)  [unwired: 2 in]
        n113 = Build Array(w347, w344, w343) -> (w346:i32[])
        n114 = To Double Precision Float(number=w346) -> (double precision float=w342:dbl[])
        n115 = case "Which ROI mode?" shown="\"PointCollection\"" w341 {
          tunnel: [w357 w360 w384] -> w329
          tunnel: [w356 w359 w383] -> w327
          tunnel: w348 -> [_ _ w382]
          tunnel: w338 -> [w357 w367 w381]
          tunnel: w343 -> [_ _ w380]
          tunnel: w342 -> [_ _ w379]
          tunnel: w340 -> [_ w369 _]
          tunnel: w339 -> [w356 w368 w378]
          tunnel: w336 -> [w358 w365 w377]
          tunnel: [w358 w364 w376] -> w335
          tunnel: [w355 w362 w375] -> w333
          tunnel: w332 -> [w355 w362 w374]
          tunnel: [_ _ w373] -> w326
          frame "none" {
          }
          frame "IMAQROIs", Default {
            w363 = TRUE ("State Changed?")
            n116 = local read "frame"() -> (w372:i32)
            n117 = property on="Image" class="ImageControl"(error in=w367) -> (error out=w360:errorcluster, "ROI"=w366:T16)  [unwired: 1 in, 1 out]
            n118 = Decrement(x=w372) -> (x-1=w371:i32)
            n119 = Replace Array Subset(array=w369, new element=w366, index=w371) -> (w370:T17)
            n120 = Bundle By Name(cluster=w365, "Data Changed?"=w363, "State Changed?"=w363) -> (w364:T2)
            n121 = Bundle By Name(cluster=w368, "ROI (frames).ROI"=w370, "last action"=last_action_enum."ROIs changed") -> (w359:T3)
          }
          frame "PointCollection" {
            n122 = case "Which tool?" shown="2" w382 {
              tunnel: w381 -> [w388 w413 w452]
              tunnel: [w388 w392 w442] -> w384
              tunnel: w378 -> [w387 w412 w451]
              tunnel: [w387 w414 w441] -> w383
              tunnel: w380 -> [_ _ _]
              tunnel: w379 -> [_ w411 w450]
              tunnel: w377 -> [w386 w395 w447]
              tunnel: [w386 w394 w446] -> w376
              tunnel: [w385 w390 w444] -> w375
              tunnel: w374 -> [w385 w391 w444]
              tunnel: [_ w389 w440] -> w373
              frame Default {
              }
              frame 1 {
                w389 = TRUE  # redraw!
                w393 = TRUE ("State Changed?")
                (unwired) 1 items=["None", "Selection Tool", "Point Tool", "Line Tool", "Rectangle Tool", "Oval Tool", "Polygon Tool", "ClosedFreehandTool", "Annulus Tool", "Rotated Rectangle Tool", "Zoom Tool", "Pan Tool", "Polyline Tool", "Freehand Tool"] ("Tool")
                n123 = call <vilib>:"Intialize Keyboard.vi"("error in (no error)"=w413) -> ("error out"=w409:errorcluster, "device ID"=w408:refnum<k1>)  [unwired: 9 in]
                n124 = call-poly <vilib>:"Acquire Input Data.vi"("device ID"=w408, "error in (no error)"=w409) -> ("device ID"=w407:refnum<k1>, "keys pressed"=w406:T21, "error out"=w410:errorcluster)  [unwired: 15 in]
                n125 = Unbundle By Name(w412) -> ("pointCollection"=w403:refnum<class "PointCollection.lvclass">)
                n126 = call-poly <vilib>:"Close Input Device.vi"("error in (no error)"=w410, "device ID"=w407) -> ("error out"=w396:errorcluster)  [unwired: 8 in]
                n127 = Search 1D Array(1D array=w406, element=T14."DELETE") -> (index of element=w404:i32)  [unwired: 1 in]
                n128 = Greater Or Equal To 0?(x=w404) -> (x >= 0?=w399:bool)
                n129 = call "find_best_match.vi"("radius"=5.0, "error in (no error)"=w396, "location (x/y/z)"=w411, "PointCollection in"=w403) -> ("error out"=w398:errorcluster, "found?"=w400:bool, "point (x/y/z)"=w401:dbl[], "PointCollection out"=w397:refnum<class "PointCollection.lvclass">)  [unwired: 4 in]
                n130 = case "Point found?" shown="True" w400 {
                  tunnel: w401 -> [_ w425]
                  tunnel: [w417 w419] -> w414
                  tunnel: w412 -> [w417 w428]
                  tunnel: w399 -> [_ w427]
                  tunnel: w398 -> [w416 w426]
                  tunnel: [w416 w421] -> w392
                  tunnel: w397 -> [_ w423]
                  tunnel: w391 -> [w415 w418]
                  tunnel: [w415 w418] -> w390
                  frame False {
                  }
                  frame True {
                    n131 = Index Array(array=w425) -> (element=w424:dbl)  [unwired: 1 in]
                    n132 = case "Delete point?" shown="False" w427 {
                      tunnel: [w432 w434] -> w420
                      tunnel: w428 -> [w431 w436]
                      tunnel: w426 -> [w430 w439]
                      tunnel: [w430 w438] -> w421
                      tunnel: w424 -> [w429 w437]
                      tunnel: w423 -> [_ w433]
                      frame False {
                        # "Insert point..."
                        n133 = Bundle By Name(cluster=w431, "selected point ID"=w429) -> (w432:T3)
                      }
                      frame True {
                        n134 = call "delete_point.vi"("error in (no error)"=w439, "point ID"=w437, "PointCollection in"=w433) -> ("error out"=w438:errorcluster, "PointCollection out"=w435:refnum<class "PointCollection.lvclass">)  [unwired: 7 in]
                        n135 = Bundle By Name(cluster=w436, "pointCollection"=w435) -> (w434:T3)
                      }
                    }
                    n136 = Bundle By Name(cluster=w420, "last action"=last_action_enum."ROIs changed") -> (w419:T3)
                  }
                }
                n137 = Bundle By Name(cluster=w395, "Data Changed?"=w393, "State Changed?"=w393) -> (w394:T2)
              }
              frame 2 {
                w440 = TRUE  # redraw!
                w443 = TRUE ("State Changed?")
                (unwired) 2 items=["None", "Selection Tool", "Point Tool", "Line Tool", "Rectangle Tool", "Oval Tool", "Polygon Tool", "ClosedFreehandTool", "Annulus Tool", "Rotated Rectangle Tool", "Zoom Tool", "Pan Tool", "Polyline Tool", "Freehand Tool"] ("Tool")
                n138 = Unbundle By Name(w451) -> ("pointCollection"=w449:refnum<class "PointCollection.lvclass">)
                n139 = call "add_point.vi"("error in (no error)"=w452, "point (x/y/z)"=w450, "PointCollection in"=w449) -> ("error out"=w442:errorcluster, "PointCollection out"=w448:refnum<class "PointCollection.lvclass">)  [unwired: 7 in]
                n140 = Bundle By Name(cluster=w447, "Data Changed?"=w443, "State Changed?"=w443) -> (w446:T2)
                n141 = Bundle By Name(cluster=w451, "last action"=last_action_enum."ROIs changed", "pointCollection"=w448) -> (w441:T3)
              }
            }
          }
        }
        n142 = case "Redraw?" shown="True" w326 {
          tunnel: [w350 w354] -> w330
          tunnel: w329 -> [w350 w353]
          tunnel: [w349 w352] -> w328
          tunnel: w327 -> [w349 w351]
          frame False {
          }
          frame True {
            n143 = call "method_redraw.vi"("Display State In"=w351, "error in (no error)"=w353) -> ("Display State Out"=w352:T3, "error out"=w354:errorcluster)  [unwired: 12 in]
          }
        }
      }
      event Data Change {
        w459 = T16 {"Global Rectangle"=[], "Contours"=[]} ("ROI")
        w463 = TRUE ("State Changed?")
        n144 = event-data() -> ()  [unwired: 1 in, 4 out]
        n145 = property on="Image" class="ImageControl"(error in=w465, "ROI"=w459) -> (error out=w455:errorcluster)  [unwired: 1 in, 1 out]
        n146 = property on="frame" class="Slide (strict)"(error in=w455, "Val(Sgnl)"=1 ("Value (Signaling)")) -> (error out=w461:errorcluster)  [unwired: 1 in, 1 out]
        n147 = call-dynamic "get_number_of_images.vi"("error in (no error)"=w461, "ImageCollection in"=w471) -> ("error out"=w458:errorcluster, "size"=w457:i32, "ImageCollection out"=w470:T13)  [unwired: 7 in]
        n148 = Bundle By Name(cluster=w467, "State Changed?"=w463, "Data Changed?"=w463) -> (w466:T2)
        n149 = Initialize Array(w459, w457) -> (w460:T17)
        n150 = Bundle By Name(cluster=w469, "number of images"=w457, "ROI (frames).ROI"=w460) -> (w468:T3)
        n151 = Greater Than 0?(x=w457) -> (x > 0?=w456:bool)
        n152 = case "Contains at least 1 image?" shown="True" w456 {
          tunnel: w458 -> [w472 w476]
          tunnel: [w472 w473] -> w464
          frame False {
          }
          frame True {
            w475 = T19."Enabled" ("Disabled")
            n153 = property on="loadROIsButton" class="Bool"(error in=w476, "DisabledEnum"=w475) -> (error out=w474:errorcluster)  [unwired: 1 in, 1 out]
            n154 = property on="showHeaderButton" class="Bool"(error in=w474, "DisabledEnum"=w475) -> (error out=w473:errorcluster)  [unwired: 1 in, 1 out]
          }
        }
      }
      event Display State Change {
        n155 = event-data() -> ()  [unwired: 1 in, 1 out]
        n156 = Unbundle By Name(w497) -> ("Refnum"=w496:refnum<vi>)
        n157 = Unbundle By Name(w479) -> ("PlotAreaSize"=w491:cluster{"Width":u32, "Height":u32})
        n158 = Not Equal?(x=cluster{"Width":u32, "Height":u32} {"Width"=0, "Height"=0} ("PlotAreaSize"), y=w491) -> (x != y?=w492:bool)
        n159 = case "new size is NOT zero?" shown="True" w492 {
          tunnel: w496 -> [_ w503]
          tunnel: w491 -> [_ w502]
          tunnel: w495 -> [w499 w501]
          tunnel: [w499 w500] -> w494
          frame False {
          }
          frame True {
            # "write new size"
            n160 = property class="Ctl"(reference=w503, error in=w501, "Container Bounds"=w502) -> (error out=w500:errorcluster)  [unwired: 1 out]
          }
        }
        n161 = Unbundle By Name(w479) -> ("ROI Tool Buttons Visible"=w490:T15, "ROI color"=w484:u32)
        n162 = call <vilib>:"Color to RGB.vi"("Color"=w484) -> ("R"=w486:u8, "G"=w487:u8, "B"=w488:u8)  [unwired: 1 out]
        n163 = Build Array(w486, w487, w488) -> (w489:u8[])
        n164 = Array To Cluster(array=w489) -> (cluster=w485:cluster{"[0]":u8, "[1]":u8, "[2]":u8})
        n165 = property on="Image" class="ImageControl"(error in=w494, "ROI Tool Buttons Visible"=w490, "ROI Color"=w485) -> (error out=w480:errorcluster)  [unwired: 1 in, 1 out]
        n166 = call "method_redraw.vi"("Display State In"=w479, "error in (no error)"=w480) -> ("Display State Out"=w477:T3, "error out"=w478:errorcluster)  [unwired: 12 in]
      }
      event Direction Change {
        # "The direction of the XControl changed from a control to an indicator or vice versa. Update the appearance accordingly."
        n167 = event-data() -> ()  [unwired: 1 in, 4 out]
        n168 = Unbundle By Name(w513) -> ("Indicator?"=w508:bool)
        n169 = Not(x=w508) -> (.not. x?=w509:bool)
        n170 = property on="loadImageButton" class="Bool"(error in=w507, "Visible"=w509) -> (error out=w506:errorcluster)  [unwired: 1 in, 1 out]
      }
      event Panel Resize {
        # "initialize area size"
        n171 = event-data() -> ("OldBnds"=w576:T22, "NewBnds"=w575:T22)  [unwired: 1 in]
        n172 = Unbundle By Name(w525) -> ("Refnum"=w522:refnum<vi>)
        n173 = property class="Ctl"(reference=w522, error in=w524) -> (error out=w523:errorcluster, "Container Bounds"=w519:T23)  [unwired: 1 out]
        n174 = Bundle By Name(cluster=w521, "PlotAreaSize"=w519) -> (w520:T3)
        n175 = Unbundle By Name(w576) -> ("right"=w573:i16, "bottom"=w572:i16)
        n176 = Unbundle By Name(w575) -> ("right"=w574:i16, "bottom"=w571:i16)
        n177 = property on="Image" class="ImageControl"(error in=w523) -> (error out=w570:errorcluster, "Image Area Height"=w566:u32, "Image Area Width"=w569:u32)  [unwired: 1 in, 1 out]
        n178 = Subtract(x=w574, y=w573) -> (x-y=w555:i16)
        n179 = Subtract(x=w571, y=w572) -> (x-y=w565:i16)
        n180 = To Unsigned Long Integer(number=w555) -> (unsigned 32bit integer=w527:u32)
        n181 = Add(x=w527, y=w569) -> (x+y=w568:u32)
        n182 = To Unsigned Long Integer(number=w565) -> (unsigned 32bit integer=w526:u32)
        n183 = Add(x=w526, y=w566) -> (x+y=w567:u32)
        n184 = property on="Image" class="ImageControl"(error in=w570, "Image Area Height"=w567, "Image Area Width"=w568) -> (error out=w564:errorcluster)  [unwired: 1 in, 1 out]
        n185 = To Long Integer(number=w555) -> (32bit integer=w533:i32)
        n186 = Bundle By Name(cluster=w517, "State Changed?"=TRUE ("Data Changed?")) -> (w516:T2)
        n187 = property on="frame" class="Slide (strict)"(error in=w564) -> (error out=w563:errorcluster, "Height"=w562:u32)  [unwired: 1 in, 1 out]
        n188 = Add(x=w526, y=w562) -> (x+y=w561:u32)
        n189 = property on="frame" class="Slide (strict)"(error in=w563, "Height"=w561) -> (error out=w558:errorcluster)  [unwired: 1 in, 1 out]
        n190 = To Long Integer(number=w526) -> (32bit integer=w556:i32)
        n191 = property on="showHeaderButton" class="Bool"(error in=w558) -> (error out=w559:errorcluster, "Top"=w560:i32)  [unwired: 1 in, 1 out]
        n192 = Add(x=w556, y=w560) -> (x+y=w557:i32)
        n193 = property on="showHeaderButton" class="Bool"(error in=w559, "Top"=w557) -> (error out=w529:errorcluster)  [unwired: 1 in, 1 out]
        n194 = property on="progress bar" class="Slide (strict)"(error in=w529) -> (error out=w530:errorcluster, "Width"=w532:u32)  [unwired: 1 in, 1 out]
        n195 = Add(x=w527, y=w532) -> (x+y=w531:u32)
        n196 = property on="progress bar" class="Slide (strict)"(error in=w530, "Width"=w531) -> (error out=w528:errorcluster)  [unwired: 1 in, 1 out]
        n197 = property on="loadPointsButton" class="Bool"(error in=w528) -> (error out=w553:errorcluster, "Left"=w554:i32)  [unwired: 1 in, 1 out]
        n198 = property on="savePointsButton" class="Bool"(error in=w528) -> (error out=w547:errorcluster, "Left"=w550:i32)  [unwired: 1 in, 1 out]
        n199 = property on="loadROIsButton" class="Bool"(error in=w528) -> (error out=w546:errorcluster, "Left"=w549:i32)  [unwired: 1 in, 1 out]
        n200 = property on="saveROIsButton" class="Bool"(error in=w528) -> (error out=w539:errorcluster, "Left"=w540:i32)  [unwired: 1 in, 1 out]
        n201 = property on="loadImageButton" class="Bool"(error in=w528) -> (error out=w535:errorcluster, "Left"=w537:i32)  [unwired: 1 in, 1 out]
        n202 = Add(x=w533, y=w554) -> (x+y=w552:i32)
        n203 = Add(x=w533, y=w550) -> (x+y=w551:i32)
        n204 = Add(x=w533, y=w549) -> (x+y=w548:i32)
        n205 = Add(x=w533, y=w540) -> (x+y=w541:i32)
        n206 = Add(x=w533, y=w537) -> (x+y=w536:i32)
        n207 = property on="loadPointsButton" class="Bool"(error in=w553, "Left"=w552) -> (error out=w545:errorcluster)  [unwired: 1 in, 1 out]
        n208 = property on="savePointsButton" class="Bool"(error in=w547, "Left"=w551) -> (error out=w543:errorcluster)  [unwired: 1 in, 1 out]
        n209 = property on="loadROIsButton" class="Bool"(error in=w546, "Left"=w548) -> (error out=w542:errorcluster)  [unwired: 1 in, 1 out]
        n210 = property on="saveROIsButton" class="Bool"(error in=w539, "Left"=w541) -> (error out=w538:errorcluster)  [unwired: 1 in, 1 out]
        n211 = property on="loadImageButton" class="Bool"(error in=w535, "Left"=w536) -> (error out=w534:errorcluster)  [unwired: 1 in, 1 out]
        n212 = Merge Errors(w545, w543, w542, w538, w534) -> (w544:errorcluster)
      }
      event Exec State Change {
        w595 = T19."Disabled and Grayed Out" ("Disabled")
        # "initialize area size"
        # "The VI owning the XControl changed from Edit Mode  to Run Mode or vice versa.\nUpdate the appearance accordingly."
        # "Handle Edit Mode & Run Mode\ncase differently"
        n213 = event-data() -> ()  [unwired: 1 in, 1 out]
        n214 = call-dynamic "destroy.vi"("error in (no error)"=w580, "ImageCollection in"=w581) -> ("error out"=w579:errorcluster)  [unwired: 8 in, 1 out]
        n215 = Unbundle By Name(w609) -> ("Run Mode?"=w604:bool, "Refnum"=w591:refnum<vi>)
        n216 = Not(x=w604) -> (.not. x?=w598:bool)
        n217 = property on="frame" class="Slide (strict)"(error in=w579, "Visible"=w598) -> (error out=w599:errorcluster)  [unwired: 1 in, 1 out]
        n218 = property on="progress bar" class="Slide (strict)"(error in=w599, "Visible"=w598) -> (error out=w597:errorcluster)  [unwired: 1 in, 1 out]
        n219 = property on="Image" class="ImageControl"(error in=w597, "ROI"=T16 {"Global Rectangle"=[], "Contours"=[]}) -> (error out=w590:errorcluster)  [unwired: 1 in, 1 out]
        n220 = property class="Ctl"(reference=w591, error in=w590) -> (error out=w578:errorcluster, "Container Bounds"=w589:T23)  [unwired: 1 out]
        n221 = Bundle By Name(cluster=T3 {"current frame index"=0, "number of images"=0, "ROI (frames)"={"ROI"=[]}, "control refs"={"frame"=refnum, "image"=refnum, "saveROIsButton"=refnum, "loadImageSwitch"=refnum, "loadROIsSwitch"=refnum, "saveROIsSwitch"=refnum, "loadImagePath"=refnum, "loadROIPath"=refnum, "redraw"=refnum}, "calibration"={"x"=0.0, "y"=0.0, "x unit"=enum."um", "y unit"=enum."um"}, "xpaths"={"x offset"="", "y offset"="", "z offset"=""}, "offset"=refnum, "XML description"="", "number of ROIs"=0.0, "ROI Tool Buttons Visible"={"Zoom Tool"=FALSE, "Selection Tool"=FALSE, "Pan Tool"=FALSE, "Point Tool"=FALSE, "Line Tool"=FALSE, "Rectangle Tool"=FALSE, "Rotated Rectangle Tool"=FALSE, "Polyline Tool"=FALSE, "Polygon Tool"=FALSE, "Freehand Tool"=FALSE, "Closed Freehand Tool"=FALSE, "Ellipse Tool"=FALSE, "Annulus Tool"=FALSE}, "ROI color"=0, "enable ROI numbering?"=FALSE, "selected path to save ROIs"=path "", "starting path"=path "", "loaded image path"=path "", "array of overlays"=[], "pointCollection"=refnum, "ROImode"=enum."none", "selected point ID"=0.0, "point radius"=0, "point colours"=[], "PlotAreaSize"={"Width"=0, "Height"=0}, "last action"=enum."not specified"} ("State"), "control refs"=w585, "ROI Tool Buttons Visible"=T15 {"Zoom Tool"=TRUE, "Selection Tool"=TRUE, "Pan Tool"=TRUE, "Point Tool"=TRUE, "Line Tool"=TRUE, "Rectangle Tool"=TRUE, "Rotated Rectangle Tool"=TRUE, "Polyline Tool"=TRUE, "Polygon Tool"=TRUE, "Freehand Tool"=TRUE, "Closed Freehand Tool"=TRUE, "Ellipse Tool"=TRUE, "Annulus Tool"=FALSE}, "point radius"=5, "PlotAreaSize"=w589) -> (w608:T3)
        n222 = Bundle By Name(cluster=w606, "State Changed?"=TRUE) -> (w605:T2)
        n223 = local write "Image"(T1 refnum ("Image")) -> ()
        n224 = property on="loadROIsButton" class="Bool"(error in=w578, "DisabledEnum"=w595) -> (error out=w601:errorcluster)  [unwired: 1 in, 1 out]
        n225 = property on="saveROIsButton" class="Bool"(error in=w601, "DisabledEnum"=w595) -> (error out=w596:errorcluster)  [unwired: 1 in, 1 out]
        n226 = property on="showHeaderButton" class="Bool"(error in=w596, "DisabledEnum"=w595) -> (error out=w593:errorcluster)  [unwired: 1 in, 1 out]
        n227 = property on="loadPointsButton" class="Bool"(error in=w593, "DisabledEnum"=w595) -> (error out=w594:errorcluster)  [unwired: 1 in, 1 out]
        n228 = property on="savePointsButton" class="Bool"(error in=w594, "DisabledEnum"=w595) -> (error out=w592:errorcluster)  [unwired: 1 in, 1 out]
        "progress bar" <- u8 0 ("progress bar")
      }
    }
    "event case no." <- w25
    n229 = Wait (ms)(milliseconds to wait=u32 0) -> ()  [unwired: 1 out]
    n230 = call "conditional_error_clearer.vi"("error in (no error)"=w30, "array of clearable error codes"=w29) -> ("error out"=w31:errorcluster)  [unwired: 9 in]
    n231 = Unbundle By Name(w31) -> ("status"=w33:bool)
    n232 = Or(x=w33, y=w35) -> (x .or. y?=w34:bool)
  }
  "Display State Out" <- w19
  "Data Out" <- w22
  "Action" <- w18
  n233 = call <vilib>:"Simple Error Handler.vi"("error in (no error)"=w15) -> ("error out"=→"error out":errorcluster)  [unwired: 4 in, 4 out]
